vi "Pump Inject.vi"(6 "auto_switch_valve":bool=TRUE, 8 "error in (no error)":errorcluster, 11 "Application in":refnum<class "Application.lvclass">) -> (0 "error out":errorcluster, 3 "Application out":refnum<class "Application.lvclass">)   [LabVIEW 2018, in "Application.lvlib" / "Application.lvclass"]
uses:
  Application.lvclass
  Application.lvclass/Application.ctl
  Hardware/cetoni Messages/Run Infuse Msg/Run Inject Msg.lvclass/Run Inject Msg.ctl
  <vilib>/ActorFramework/Message Enqueuer/Message Enqueuer.lvclass/Message Enqueuer.ctl
  <vilib>/ActorFramework/Message Enqueuer/Enqueue.vi
  Hardware/cetoni Messages/Run Infuse Msg/Run Inject Msg.lvclass
  C:/Program Files/National Instruments/LabVIEW 2018/vi.lib/ActorFramework/Message/Message.lvclass
  <vilib>/ActorFramework/Message Priority Queue/Priority Enqueue.vi
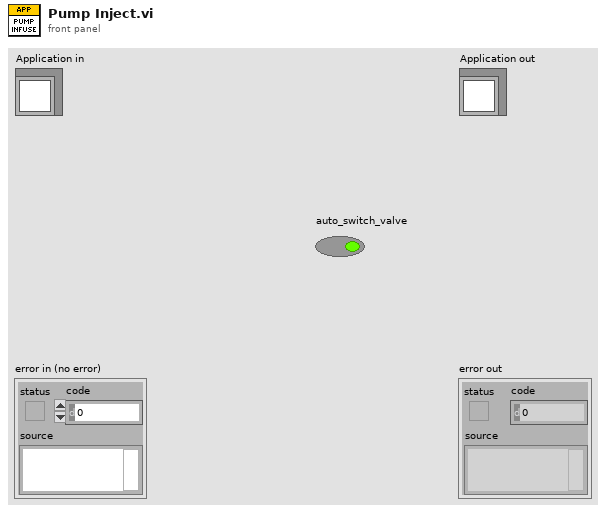
[diagram p1: front panel]
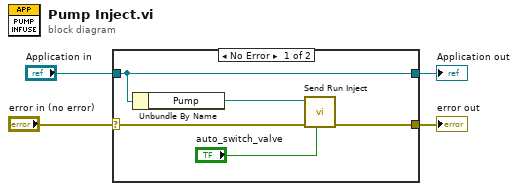
[diagram p0: block diagram]
diagram:
  n1 = case shown="No Error" "error in (no error)" {
    selector: "error in (no error)" -> [w7 w11]
    tunnel: [w6 w11] -> w3
    tunnel: [w9 w10] -> w1
    tunnel: "Application in" -> [w9 w10]
    frame No Error {
      n2 = Unbundle By Name(w9) -> ("Pump"=w8:refnum<class "Message Enqueuer.lvclass">)
      n3 = call "Send Run Inject.vi"("auto_switch_valve"="auto_switch_valve", "error in (no error)"=w7, "Message Enqueuer"=w8) -> ("error out"=w6:errorcluster)  [unwired: 7 in, 1 out]
    }
    frame Error {
    }
  }
  "error out" <- w3
  "Application out" <- w1
